vi "Destroy.vi"(0 "reference":refnum<class "CallEdge.lvclass">, 5 "error in (no error)":errorcluster) -> (15 "# of objects":i32, 19 "error out":errorcluster)   [LabVIEW 2012, in "CallEdge.lvclass"]
doc: "Destroys a CallEdge object created with a CallEdge constructor VI.\n\n[GOOP 2.3]"
uses:
  <resource>/Framework/Providers/Open_GDS/UML/CallEdge_class/CallEdge.lvclass
  <resource>/Framework/Providers/Open_GDS/UML/SegmentedLineEdge_class/SegmentedLineEdge.lvclass
panel:
  out "reference out":refnum<class "CallEdge.lvclass">
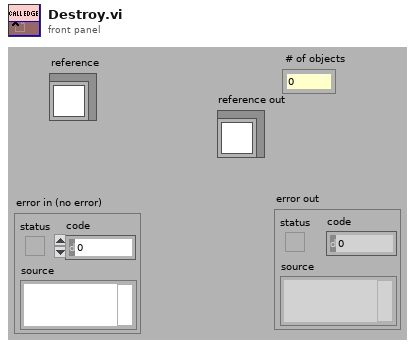
[diagram p1: front panel]
types:
  T1 = typedef "CallEdge.lvclass/ObjectAttributes.ctl" = cluster{"signal":bool}
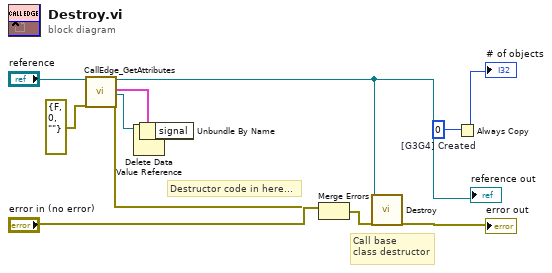
[diagram p0: block diagram]
diagram:
  w1 = 0  # [G3G4] Created
  # "Call base\nclass destructor"
  # "Destructor code in here..."
  n1 = call <resource>:"CallEdge_GetAttributes.vi"("reference in"="reference", "error in (no error)"=errorcluster {"status"=FALSE, "code"=0, "source"=""}) -> ("reference out"=w6:refnum<class "CallEdge.lvclass">, "Data"=w4:T1, "DataRef"=w3:refnum<data-value>, "error out"=w7:errorcluster)  [unwired: 1 in, 13 out]
  "reference out" <- w6
  n2 = Delete Data Value Reference(data value reference=w3) -> ()  [unwired: 1 in, 2 out]
  n3 = Unbundle By Name(w4) -> ()  [unwired: 1 out]
  n4 = Merge Errors("error in (no error)", w7) -> (w5:errorcluster)
  n5 = call-parent "Destroy.vi"("reference"=w6, "error in (no error)"=w5) -> ("error out"=→"error out":errorcluster)  [unwired: 16 in, 1 out]
  n6 = Always Copy(1:w1) -> (0:→"# of objects":i32)
